vi "Simple DMM Scan PRD 32 - Loop.vi"() -> ()   [LabVIEW 2021]
uses:
  DMM SCAN PRD 32V-16C/Typedefs/Scan configuration.ctl
  <instrlib>/niDMM/nidmm.llb/niDMM Resolution in Digits.ctl
  DMM SCAN PRD 32V-16C/Typedefs/Formatted measurement.ctl
  DMM SCAN PRD 32V-16C/Typedefs/Scan Resource Names.ctl
  DMM SCAN PRD 32V-16C/DMM_Scan PXI RLY Driver 32V-16C.lvlib
panel:
  out "Total Scan Time (s)":dbl=0.3051954999998543 format="%#.3p"
  in  "stop":bool
  out "Formatted Measurements":T1[](array[typedef])=[{"Channel"="ch0", "Switch Time"=0.03294069999992644, "Formatted Measurement"="9.89152V (dc)", "Out of Range"=FALSE}, {"Channel"="ch1", "Switch Time"=0.03199610000001485, "Formatted Measurement"="96.9794mV (dc)", "Out of Range"=FALSE}, {"Channel"="ch32", "Switch Time"=0.24025400000004993, "Formatted Measurement"="9.379824uA (dc)", "Out of Range"=FALSE}] {"Switch Time" format="%#_3p"}
  in  "Scan Configuration":T2[](array[typedef])=[{"Channel"="ch0", "Resolution in Digits"=5.5, "Range and Function"=enum."DC 10 V"}, {"Channel"="ch1", "Resolution in Digits"=5.5, "Range and Function"=enum."DC 100 mV"}, {"Channel"="ch32", "Resolution in Digits"=6.5, "Range and Function"=enum."DC 10 uA"}] {"Resolution in Digits" items=["3 1/2"=3.5, "4 1/2"=4.5, "5 1/2"=5.5, "6 1/2"=6.5, "7 1/2"=7.5]}
  out "error out":errorcluster
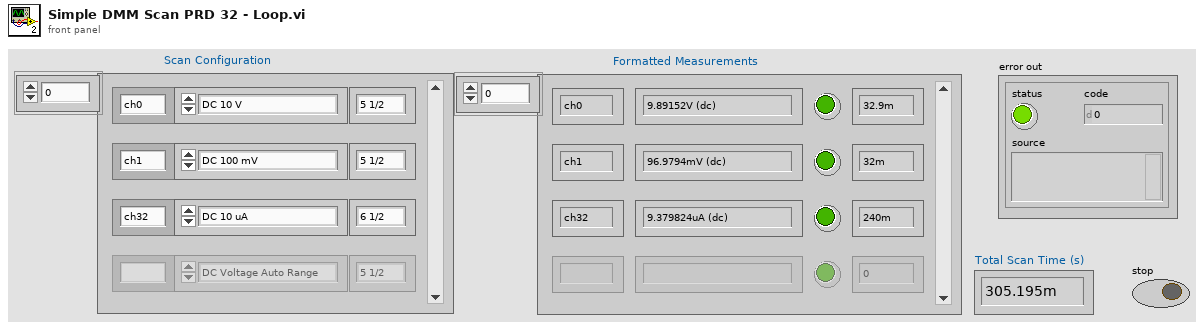
[diagram p1: front panel]
types:
  T1 = typedef "DMM_Scan PXI RLY Driver 32V-16C.lvlib/Formatted measurement.ctl" = cluster{"Channel":string, "Switch Time":dbl, "Formatted Measurement":string, "Out of Range":bool}
  T2 = typedef "DMM_Scan PXI RLY Driver 32V-16C.lvlib/Scan configuration.ctl" = cluster{"Channel":string, "Resolution in Digits":T3, "Range and Function":enum16{"DC Voltage Auto Range", "DC 100 mV", "DC 1 V ", "DC 10 V", "DC 100 V", "DC 300 V", " ", "AC Voltage Auto Range", "AC 50 mV", "AC 200 mV", "AC 500 mV", "AC 2 V", "AC 5 V", "AC 20 V", "AC 50 V", "AC 300 V", "  ", "DC Current Auto Range", "DC 1 uA", "DC 10 uA", "DC 100 uA", "DC 1 mA", "DC 10 mA", "DC 20 mA", "DC 100 mA", "DC 200 mA", "DC 1 A", "DC 3 A", "   ", "AC Current Auto Range", "AC 100 uA", "AC 1 mA", "AC 10 mA", "AC 100 mA", "AC 500 mA", "AC 1 A", "AC 3 A", "    ", "Resistance Auto Range", "Res 100 Ohm", "Res 1 kOhm", "Res 10 kOhm", "Res 100 kOhm", "Res 1 MOhm", "Res 10 MOhm", "Res 100 MOhm", "Res 5 GOhm", "     ", "Frequency AC Auto Range", "Freq AC 50 mV", "Freq AC 500 mV", "Freq AC 5 V", "Freq AC 50 V", "Freq AC 300 V", "      ", "Period AC Auto Range", "Period AC 50 mV", "Period AC 500 mV", "Period AC 5 V", "Period AC 50 V", "Period AC 300 V"}}
  T3 = typedef "niDMM Resolution in Digits.ctl" = dbl
  T4 = typedef "DMM_Scan PXI RLY Driver 32V-16C.lvlib/Scan Resource Names.ctl" = cluster{"DMM Resource Name":refnum<k15>, "MUX and Shunt Resource Name":refnum<k15>}
  T5 = typedef "DMM_Scan PXI RLY Driver 32V-16C.lvlib/Scan Resource Handles Out.ctl" = cluster{"DMM Handle":refnum<k15>, "MUX Handle":refnum<k15>, "Relays Debounce Time (ms)":u32, "Close all Shunts?":bool}
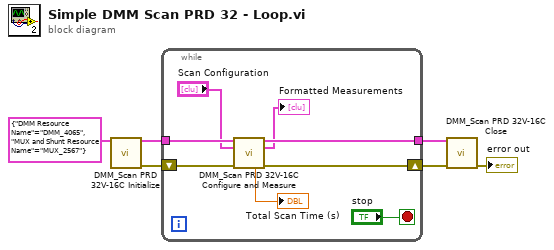
[diagram p0: block diagram]
diagram:
  n1 = call "DMM_Scan PRD 32V-16C Initialize.vi"("Scan Resource Names"=T4 {"DMM Resource Name"="DMM_4065", "MUX and Shunt Resource Name"="MUX_2567"} ("Scan Resources Names")) -> ("Scan Resource Handles out"=w3:T5, "error out"=w6:errorcluster)  [unwired: 12 in, 1 out]
  n2 = while {
    tunnel: w3 -> [w12]
    tunnel: [w11] -> w2
    shift-right: [w13] -> w5
    shift-left: w6 -> [w14]
    stop <- "stop" stop-if-true
    n3 = call "DMM_Scan PRD 32V-16C Configure and Measure.vi"("Scan Resources Handles In"=w12, "Scan Configuration"="Scan Configuration", "error in"=w14) -> ("Scan Resources Handles Out"=w11:T5, "Formatted Measurements"=→"Formatted Measurements":T1[], "Total Scan Time (s)"=→"Total Scan Time (s)":dbl, "error out"=w13:errorcluster)  [unwired: 7 in, 2 out]
  }
  n4 = call "DMM_Scan PRD 32V-16C Close.vi"("Scan Resources Handles In"=w2, "error in"=w5) -> ("error out"=→"error out":errorcluster)  [unwired: 13 in]
